vi "Deviation.vi"(0 "voltage RMS values":dbl[](array[numeric]), 9 "system info in":refnum<class "EP System Info.lvclass">, 11 "error in (no error)":errorcluster) -> (4 "Urms-under [V]":dbl[](array[numeric]), 6 "Urms-over [V]":dbl[](array[numeric]), 10 "system info out":refnum<class "EP System Info.lvclass">, 15 "error out":errorcluster)   [LabVIEW 2014, in "NI_EP_Power Quality.lvlib"]
doc: "Calculates underdeviation and overdeviation values from 10/12-cycle voltage RMS values. You can use the RMS (10 or 12 Cycles) VI to calculate voltage RMS values.\n\nThis VI supports measuring single-line and multiple-line systems."
uses:
  <vilib>/addons/Electrical Power/PQ/NI_EP_Power Quality.lvlib
  <vilib>/addons/Electrical Power/PQ/Common/Classes/System Info/EP System Info.lvclass
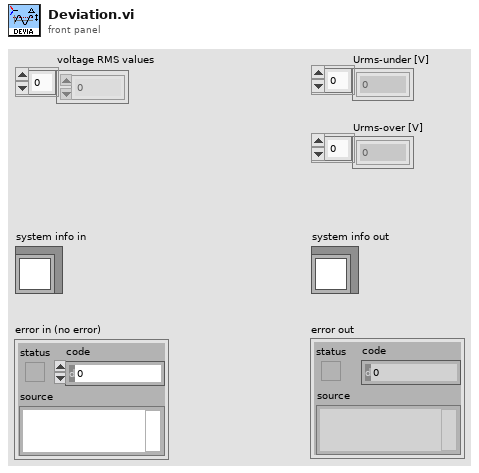
[diagram p1: front panel]
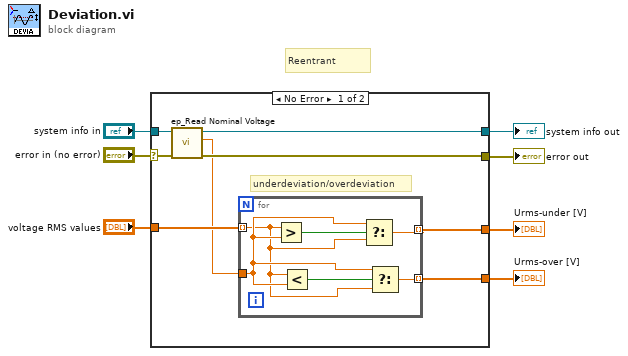
[diagram p0: block diagram]
diagram:
  # "Reentrant"
  n1 = case shown="No Error" "error in (no error)" {
    selector: "error in (no error)" -> [w13 w23]
    tunnel: [w12 w23] -> w3
    tunnel: "system info in" -> [w15 w22]
    tunnel: "voltage RMS values" -> [w11 _]
    tunnel: [w14 w22] -> w5
    tunnel: [w9 _] -> w2
    tunnel: [w8 _] -> w1
    frame No Error {
      # "underdeviation/overdeviation"
      n2 = call <vilib>:"ep_Read Nominal Voltage.vi"("error in (no error)"=w13, "system info in"=w15) -> ("error out"=w12:errorcluster, "nominal voltage [V]"=w10:dbl, "system info out"=w14:refnum<class "EP System Info.lvclass">)  [unwired: 7 in]
      n3 = for {
        tunnel: w11 -> [w16] mode=indexing
        tunnel: w10 -> [w17]
        tunnel: [w20] -> w9 mode=indexing
        tunnel: [w18] -> w8 mode=indexing
        n4 = Greater?(x=w16, y=w17) -> (0:w21:bool)
        n5 = Less?(x=w16, y=w17) -> (x < y?=w19:bool)
        n6 = Select(t=w17, s=w21, f=w16) -> (s? t:f=w20:dbl)
        n7 = Select(t=w17, s=w19, f=w16) -> (s? t:f=w18:dbl)
      }
    }
    frame Error {
    }
  }
  "system info out" <- w5
  "error out" <- w3
  "Urms-under [V]" <- w2
  "Urms-over [V]" <- w1
